vi "Pulse Timer.vi"(10 "Time":u32, 11 "Start":bool) -> (2 "Timeout":bool, 3 "Elapsed":u32)   [LabVIEW 2011]
panel:
  in  "Motor Timeout in":u32
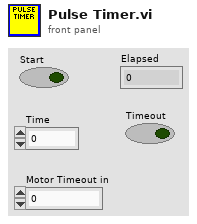
[diagram p1: front panel]
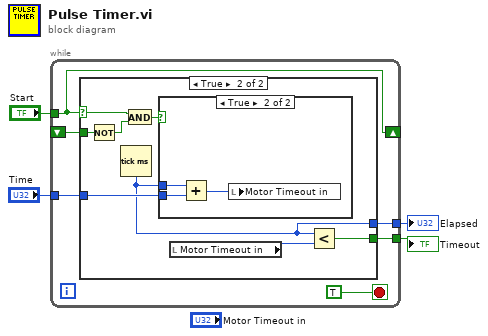
[diagram p0: block diagram]
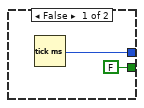
[diagram p2: hidden frame]
diagram:
  n1 = while {
    shift-right: [w5] -> _
    shift-left: _ -> [w8]
    tunnel: [w9] -> w4
    tunnel: "Start" -> [w5]
    tunnel: "Time" -> [w7]
    tunnel: [w6] -> w1
    stop <- TRUE stop-if-true
    n2 = case shown="True" w5 {
      selector: w5 -> [_ w14]
      tunnel: [FALSE w20] -> w9
      tunnel: w8 -> [_ w17]
      tunnel: w7 -> [_ w16]
      tunnel: [w11 w15] -> w6
      frame False {
        n3 = Tick Count (ms)() -> (millisecond timer value=w11:u32)
      }
      frame True {
        n4 = Not(x=w17) -> (.not. x?=w19:bool)
        n5 = Tick Count (ms)() -> (millisecond timer value=w15:u32)
        n6 = And(x=w14, y=w19) -> (x .and. y?=w18:bool)
        n7 = case shown="True" w18 {
          tunnel: w15 -> [_ w23]
          tunnel: w16 -> [_ w22]
          frame False {
          }
          frame True {
            n8 = Add(x=w23, y=w22) -> (x+y=w21:u32)
            n9 = local write "Motor Timeout in"(w21) -> ()
          }
        }
        n10 = local read "Motor Timeout in"() -> (w13:u32)
        n11 = Less?(x=w15, y=w13) -> (x < y?=w20:bool)
      }
    }
  }
  "Timeout" <- w4
  "Elapsed" <- w1
